vi "执行文件路径修正V2.vi"(1 "Path in":path) -> (0 "Path out":path)   [LabVIEW 2013]
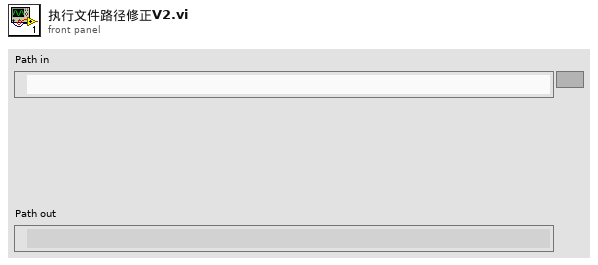
[diagram p1: front panel]
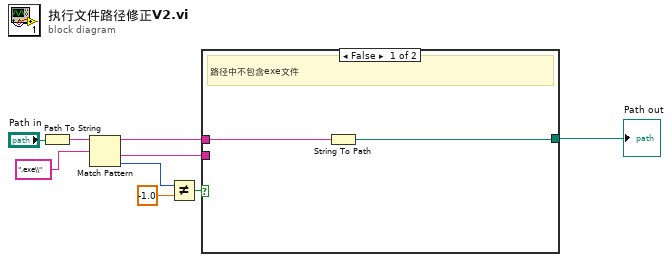
[diagram p0: block diagram]
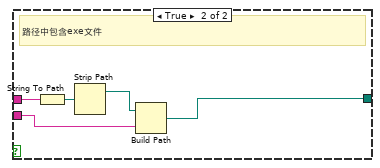
[diagram p2: hidden frame]
diagram:
  n1 = Path To String(path="Path in") -> (string=w2:string)
  n2 = Match Pattern(string=w2, regular expression=".exe\\") -> (before substring=w8:string, after substring=w7:string, offset past match=w4:i32)  [unwired: 1 in, 1 out]
  n3 = Not Equal?(x=w4, y=-1.0) -> (x != y?=w6:bool)
  n4 = case shown="False" w6 {
    tunnel: w8 -> [w11 w16]
    tunnel: w7 -> [_ w13]
    tunnel: [w10 w12] -> w3
    frame False {
      # "路径中不包含exe文件"
      n5 = String To Path(string=w11) -> (path=w10:path)
    }
    frame True {
      # "路径中包含exe文件"
      n6 = String To Path(string=w16) -> (path=w15:path)
      n7 = Strip Path(path=w15) -> (stripped path=w14:path)  [unwired: 1 out]
      n8 = Build Path(base path=w14, name or relative path=w13) -> (appended path=w12:path)
    }
  }
  "Path out" <- w3
